vi "MainPicFloatMot.vi"() -> ()   [LabVIEW 2010]
uses:
  <vilib>/Instr/_visa.llb/VISA Flush IO Buffer Mask.ctl
  Variable globale 1.vi
  <vilib>/Instr/_visa.llb/VISA Configure Serial Port (Instr).vi
panel:
  out "error out 2":errorcluster caption="sortie d'erreur"
  in  "Type":i32=138 min=138 max=139
  out "Float recu":sgl
  in  "Float envoyé":sgl=25.45
  out "Iteration 3":i32
  out "Iteration reception":i32
  out "Iteration Envoi":i32
  out "Checksum calculé":i32
  out "Checksum reçu":i32
  out "Type de donnee (ID)":i32
  out "Byte Start ?":bool
  out "Retour 2":string
  in  "stop secu":bool
  in  "STOP":bool
  out "error out":errorcluster caption="sortie d'erreur"
  in  "baud rate (9600)":u32=9600 caption="débit en bauds (9600)"
  in  "Port Com":refnum<visa-resource-name> caption="Nom de ressource VISA"
  # "Envoi"
  # "Réception"
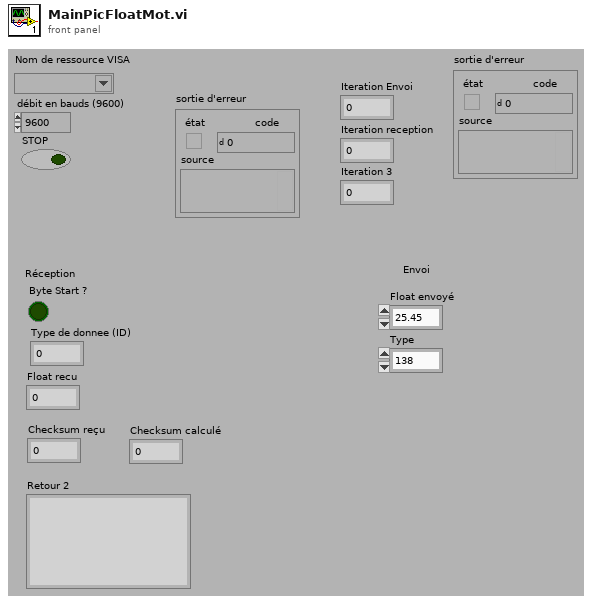
[diagram p1: front panel]
types:
  T1 = typedef "VISA Flush IO Buffer Mask.ctl" = u16
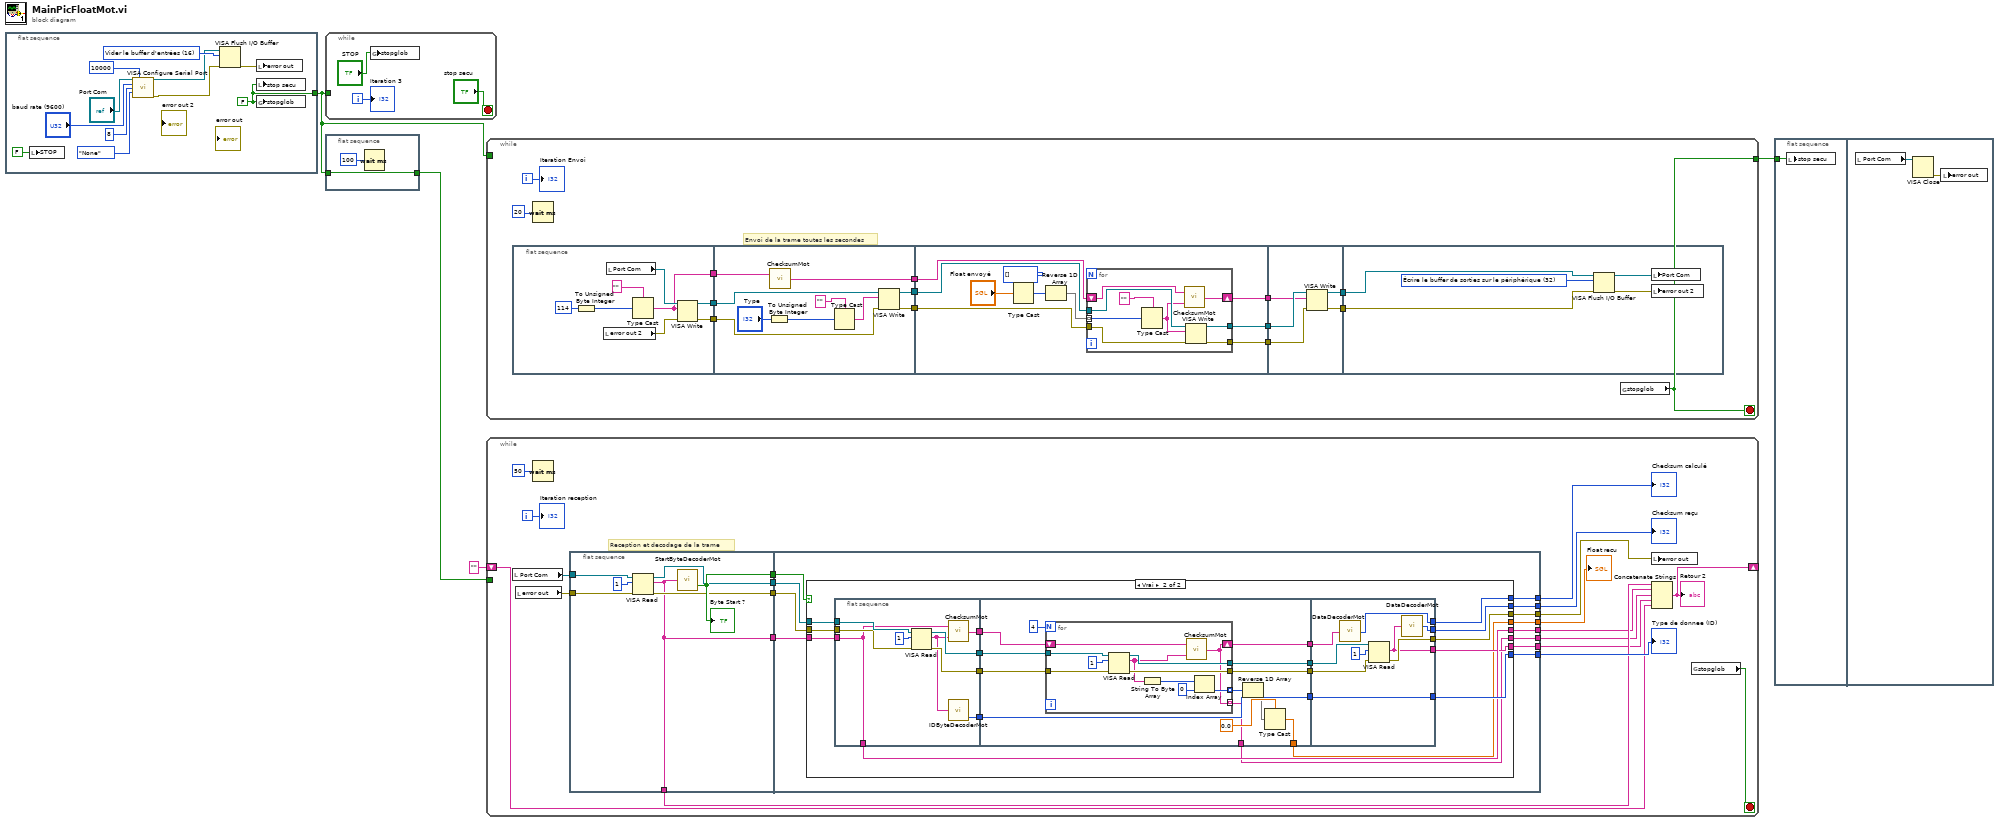
[diagram p0: block diagram]
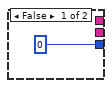
[diagram p2: hidden frame]
diagram:
  n1 = flat-sequence {
    tunnel: [w7] -> w2
    frame #0 {
      w7 = FALSE
      w10 = T1 16 items=["Vider le buffer d'entrées"=16, "Écrire le buffer de sorties sur le périphérique"=32, "Vider le buffer d'entrées (Pas d'E/S)"=64, "Vider le buffer de sorties"=128] ("Mask")
      n2 = local write "STOP"(FALSE) -> ()
      n3 = call-poly "VISA Configure Serial Port"("VISA resource name"="Port Com", "timeout (10sec)"=u32 10000, "baud rate (9600)"="baud rate (9600)", "data bits (8)"=u16 8, "parity (0:none)"=enum16{"None", "Odd", "Even", "Mark", "Space"}."None") -> ("VISA resource name out"=w6:refnum<visa-resource-name>, "error out"=w5:errorcluster)  [unwired: 9 in]
      n4 = VISA Flush I/O Buffer(VISA resource name=w6, mask (16)=w10, error in (no error)=w5) -> (error out=w8:errorcluster)  [unwired: 1 out]
      n5 = local write "error out"(w8) -> ()
      n6 = local write "stop secu"(w7) -> ()
      n7 = global write "Variable globale 1.vi" "stopglob"(w7) -> ()
    }
  }
  n8 = while {
    tunnel: w2 -> [_]
    i -> [w16]
    stop <- "stop secu" stop-if-true
    n9 = global write "Variable globale 1.vi" "stopglob"("STOP") -> ()
    "Iteration 3" <- w16
  }
  n10 = flat-sequence {
    tunnel: w2 -> [w19]
    tunnel: [w19] -> w1
    frame #0 {
      n11 = Wait (ms)(milliseconds to wait=u32 100 ("attente (ms)")) -> ()  [unwired: 1 out]
    }
  }
  n12 = while {
    tunnel: [w28] -> w4
    tunnel: w2 -> [_]
    i -> [w27]
    stop <- w28 stop-if-true
    # "Envoi de la trame toutes les secondes"
    n13 = flat-sequence {
      tunnel: [w39] -> w34
      tunnel: [w38] -> w33
      tunnel: [w37] -> w30
      tunnel: w34 -> [w52]
      tunnel: w33 -> [w51]
      tunnel: [w50] -> w32
      tunnel: [w49] -> w31
      tunnel: w30 -> [w48]
      tunnel: [w47] -> w29
      tunnel: w32 -> [w57]
      tunnel: w31 -> [w59]
      tunnel: w29 -> [w55]
      tunnel: [w58] -> w26
      tunnel: [w56] -> w25
      tunnel: [w54] -> w24
      tunnel: w26 -> [w76]
      tunnel: w25 -> [w75]
      tunnel: w24 -> [w74]
      tunnel: [w73] -> w22
      tunnel: [w72] -> w21
      tunnel: w22 -> [w81]
      tunnel: w21 -> [w80]
      frame #0 {
        n14 = To Unsigned Byte Integer(number=114) -> (unsigned 8bit integer=w36:u8)
        n15 = local read "error out 2"() -> (w35:errorcluster)
        n16 = local read "Port Com"() -> (w42:refnum<visa-resource-name>)
        n17 = Type Cast(type="", x=w36) -> (*(type *) &x=w37:string)
        n18 = VISA Write(VISA resource name=w42, write buffer=w37, error in (no error)=w35) -> (VISA resource name out=w39:refnum<visa-resource-name>, error out=w38:errorcluster)  [unwired: 1 out]
      }
      frame #1 {
        n19 = To Unsigned Byte Integer(number="Type") -> (unsigned 8bit integer=w45:u8)
        n20 = call "ChecksumMot.vi"("Byte1"=w48) -> ("chaîne"=w47:string)  [unwired: 1 in]
        n21 = Type Cast(type="", x=w45) -> (*(type *) &x=w43:string)
        n22 = VISA Write(VISA resource name=w52, write buffer=w43, error in (no error)=w51) -> (VISA resource name out=w49:refnum<visa-resource-name>, error out=w50:errorcluster)  [unwired: 1 out]
      }
      frame #2 {
        n23 = Type Cast(type=i8[] [] ("tableau d'octets non signés"), x="Float envoyé") -> (*(type *) &x=w62:i8[])
        n24 = Reverse 1D Array(array=w62) -> (reversed array=w53:i8[])
        n25 = for {
          tunnel: w53 -> [w71] mode=indexing
          tunnel: w59 -> [w69]
          tunnel: [w68] -> w58
          tunnel: w57 -> [w67]
          tunnel: [w66] -> w56
          shift-right: [w63] -> w54
          shift-left: w55 -> [w65]
          n26 = Type Cast(type="", x=w71) -> (*(type *) &x=w64:string)
          n27 = call "ChecksumMot.vi"("Byte2"=w64, "Byte1"=w65) -> ("chaîne"=w63:string)
          n28 = VISA Write(VISA resource name=w69, write buffer=w64, error in (no error)=w67) -> (VISA resource name out=w68:refnum<visa-resource-name>, error out=w66:errorcluster)  [unwired: 1 out]
        }
      }
      frame #3 {
        n29 = VISA Write(VISA resource name=w76, write buffer=w74, error in (no error)=w75) -> (VISA resource name out=w73:refnum<visa-resource-name>, error out=w72:errorcluster)  [unwired: 1 out]
      }
      frame #4 {
        w77 = T1 32 items=["Vider le buffer d'entrées"=16, "Écrire le buffer de sorties sur le périphérique"=32, "Vider le buffer d'entrées (Pas d'E/S)"=64, "Vider le buffer de sorties"=128] ("Mask")
        n30 = VISA Flush I/O Buffer(VISA resource name=w81, mask (16)=w77, error in (no error)=w80) -> (VISA resource name out=w78:refnum<visa-resource-name>, error out=w79:errorcluster)
        n31 = local write "Port Com"(w78) -> ()
        n32 = local write "error out 2"(w79) -> ()
      }
    }
    n33 = Wait (ms)(milliseconds to wait=u32 20 ("attente (ms)")) -> ()  [unwired: 1 out]
    n34 = global read "Variable globale 1.vi" "stopglob"() -> (w28:bool)
    "Iteration Envoi" <- w27
  }
  n35 = while {
    shift-right: [w85] -> _
    shift-left: "" -> [w86]
    tunnel: w1 -> [_]
    i -> [w84]
    stop <- w101 stop-if-true
    # "Reception et decodage de la trame"
    n36 = local read "Port Com"() -> (w99:refnum<visa-resource-name>)
    n37 = local read "error out"() -> (w98:errorcluster)
    n38 = Wait (ms)(milliseconds to wait=u32 50 ("attente (ms)")) -> ()  [unwired: 1 out]
    n39 = flat-sequence {
      tunnel: w99 -> [w107]
      tunnel: w98 -> [w106]
      tunnel: [w105] -> w97
      tunnel: [w104] -> w96
      tunnel: [w103] -> w95
      tunnel: [w102] -> w93
      tunnel: [w102] -> w89
      tunnel: w97 -> [w120]
      tunnel: w96 -> [w119]
      tunnel: w95 -> [w118]
      tunnel: [w117] -> w94
      tunnel: w93 -> [w116]
      tunnel: [w115] -> w92
      tunnel: [w114] -> w91
      tunnel: [w113] -> w90
      tunnel: [w112] -> w88
      tunnel: [w111] -> w87
      tunnel: [w110] -> w83
      tunnel: [w109] -> w82
      frame #0 {
        n40 = VISA Read(VISA resource name=w107, byte count=u32 1 ("nombre d'octets"), error in (no error)=w106) -> (VISA resource name out=w104:refnum<visa-resource-name>, read buffer=w102:string, error out=w103:errorcluster)  [unwired: 1 out]
        n41 = call "StartByteDecoderMot.vi"("byte1"=w102) -> ("Byte Start ?"=w105:bool)  [unwired: 1 in]
        "Byte Start ?" <- w105
      }
      frame #1 {
        n42 = case shown="Vrai" w120 {
          tunnel: w119 -> [_ w140]
          tunnel: w118 -> [_ w139]
          tunnel: [0 ("Type de donnee (ID)") w138] -> w117
          tunnel: w116 -> [_ w133]
          tunnel: [_ w131] -> w115
          tunnel: [_ w130] -> w114
          tunnel: [_ w129] -> w113
          tunnel: [_ w128] -> w112
          tunnel: [_ w127] -> w111
          tunnel: [_ w124] -> w110
          tunnel: [_ w122] -> w109
          frame False {
          }
          frame True {
            n43 = flat-sequence {
              tunnel: w140 -> [w149]
              tunnel: w139 -> [w148]
              tunnel: [w146] -> w137
              tunnel: [w145] -> w136
              tunnel: [w144] -> w135
              tunnel: w133 -> [w141]
              tunnel: [w142] -> w132
              tunnel: [w141] -> w128
              tunnel: w137 -> [w162]
              tunnel: w136 -> [w161]
              tunnel: w135 -> [w158]
              tunnel: [w162] -> w134
              tunnel: w132 -> [w154]
              tunnel: [w160] -> w126
              tunnel: [w159] -> w125
              tunnel: [w155] -> w124
              tunnel: [w153] -> w123
              tunnel: [w151] -> w122
              tunnel: [w182] -> w138
              tunnel: w134 -> [w182]
              tunnel: [w180] -> w131
              tunnel: [w179] -> w130
              tunnel: [w178] -> w129
              tunnel: [w177] -> w127
              tunnel: w126 -> [w176]
              tunnel: w125 -> [w175]
              tunnel: w123 -> [w174]
              frame #0 {
                n44 = VISA Read(VISA resource name=w149, byte count=u32 1 ("nombre d'octets"), error in (no error)=w148) -> (VISA resource name out=w145:refnum<visa-resource-name>, read buffer=w143:string, error out=w144:errorcluster)  [unwired: 1 out]
                n45 = call "ChecksumMot.vi"("Byte2"=w143, "Byte1"=w141) -> ("chaîne"=w142:string)
                n46 = call "IDByteDecoderMot.vi"("byte1"=w143) -> ("Type de donnee (ID)"=w146:i32)  [unwired: 2 out]
              }
              frame #1 {
                n47 = for {
                  N: 4 -> [_]
                  tunnel: w161 -> [w172]
                  tunnel: [w171] -> w160
                  tunnel: [w170] -> w159
                  tunnel: w158 -> [w169]
                  tunnel: [w166] -> w156 mode=indexing
                  shift-right: [w163] -> w153
                  shift-left: w154 -> [w165]
                  tunnel: [w163] -> w151 mode=indexing
                  n48 = VISA Read(VISA resource name=w172, byte count=u32 1 ("nombre d'octets"), error in (no error)=w169) -> (VISA resource name out=w171:refnum<visa-resource-name>, read buffer=w164:string, error out=w170:errorcluster)  [unwired: 1 out]
                  n49 = String To Byte Array(string=w164) -> (unsigned byte array=w168:u8[])
                  n50 = call "ChecksumMot.vi"("Byte2"=w164, "Byte1"=w165) -> ("chaîne"=w163:string)
                  n51 = Index Array(array=w168, index=0 ("indice")) -> (element=w166:u8)
                }
                n52 = Reverse 1D Array(array=w156) -> (reversed array=w150:u8[])
                n53 = Type Cast(type=sgl 0.0, x=w150) -> (*(type *) &x=w155:sgl)
              }
              frame #2 {
                n54 = call "DataDecoderMot.vi"("byte1"=w174) -> ("Data"=w180:i32)
                n55 = VISA Read(VISA resource name=w176, byte count=u32 1 ("nombre d'octets"), error in (no error)=w175) -> (read buffer=w177:string, error out=w178:errorcluster)  [unwired: 2 out]
                n56 = call "DataDecoderMot.vi"("byte1"=w177) -> ("Data"=w179:i32)
              }
            }
          }
        }
      }
    }
    n57 = local write "error out"(w90) -> ()
    n58 = Concatenate Strings(w89, w88, w82, w87, w86) -> (w85:string)
    "Retour 2" <- w85
    n59 = global read "Variable globale 1.vi" "stopglob"() -> (w101:bool)
    "Type de donnee (ID)" <- w94
    "Checksum reçu" <- w91
    "Checksum calculé" <- w92
    "Iteration reception" <- w84
    "Float recu" <- w83
  }
  n60 = flat-sequence {
    tunnel: w4 -> [w183]
    frame #0 {
      n61 = local write "stop secu"(w183) -> ()
    }
    frame #1 {
      n62 = local read "Port Com"() -> (w185:refnum<visa-resource-name>)
      n63 = VISA Close(VISA resource name=w185) -> (error out=w184:errorcluster)  [unwired: 1 in]
      n64 = local write "error out"(w184) -> ()
    }
  }
